vi "2DUniqueArraySet.vi"(10 "Colums":i32=6, 11 "Rows":i32=3) -> (0 "2D Double Array":i32[][](array[numeric]), 3 "2D String Array":string[][](array[string]))   [LabVIEW 2023]
uses:
  <vilib>/numeric/Random Number (Range) U64.vi
  <vilib>/numeric/sub_Random U32.vi
panel:
  # "Генерира 6 \"уникални\" числа.\n\"Унникалността\" се запазва единствено и само за елементите в колоните на даден ред,\n но не и между редовете."
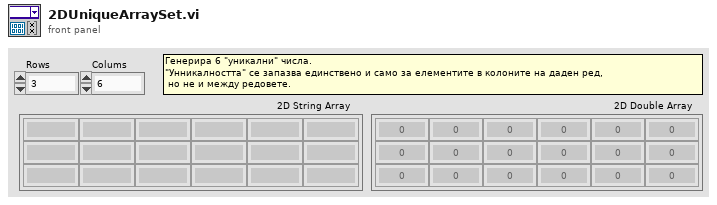
[diagram p1: front panel]
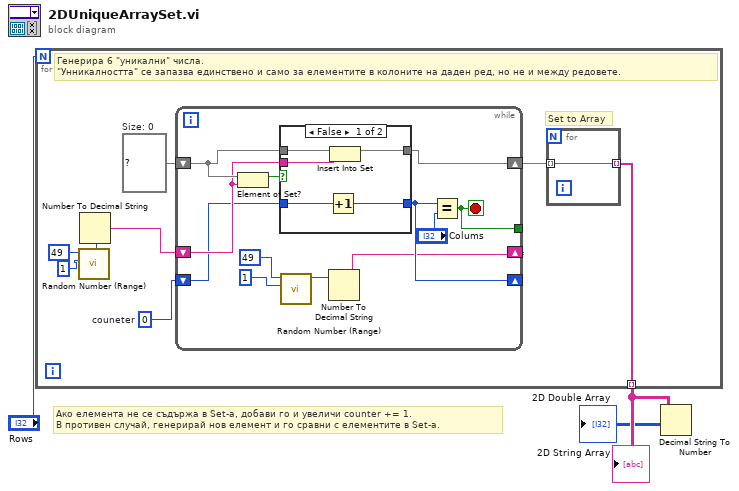
[diagram p0: block diagram]
diagram:
  # "Ако елемента не се съдържа в Set-а, добави го и увеличи counter += 1.\nВ противен случай, генерирай нов елемент и го сравни с елементите в Set-а."
  n1 = for {
    N: "Rows" -> [_]
    tunnel: [w5] -> w2 mode=indexing
    w4 = set{string} {}  # Size: 0
    w7 = 0  # couneter
    # "Генерира 6 \"уникални\" числа.\n\"Унникалността\" се запазва единствено и само за елементите в колоните на даден ред, но не и между редовете."
    # "Set to Array"
    n2 = call-poly <vilib>:"Random Number (Range).vi"("lower bound (0)"=u64 1, "upper bound (100)"=u64 49) -> ("number"=w11:u64)  [unwired: 9 in]
    n3 = Number To Decimal String(number=w11) -> (decimal integer string=w8:string)  [unwired: 1 in]
    n4 = while {
      shift-right: [w21] -> w6
      shift-left: w4 -> [w23]
      shift-right: [w14] -> _
      shift-left: w8 -> [w22]
      shift-right: [w19] -> _
      shift-left: w7 -> [w20]
      tunnel: [w13] -> _
      stop <- w13 stop-if-true
      n5 = Element of Set?(10:w22, 11:w23) -> (3:w24:bool)
      n6 = case shown="False" w24 {
        tunnel: w23 -> [w29 w31]
        tunnel: w22 -> [w27 _]
        tunnel: [w28 w31] -> w21
        tunnel: w20 -> [w26 w30]
        tunnel: [w25 w30] -> w19
        frame False {
          n7 = Increment(x=w26) -> (x+1=w25:i32)
          n8 = Insert Into Set(10:w27, 11:w29) -> (3:w28:set{string})  [unwired: 1 out]
        }
        frame True {
        }
      }
      n9 = call-poly <vilib>:"Random Number (Range).vi"("lower bound (0)"=u64 1, "upper bound (100)"=u64 49) -> ("number"=w17:u64)  [unwired: 9 in]
      n10 = Number To Decimal String(number=w17) -> (decimal integer string=w14:string)  [unwired: 1 in]
      n11 = Equal?(x=w19, y="Colums") -> (x = y?=w13:bool)
    }
    n12 = for {
      tunnel: [w12] -> w5 mode=indexing
      tunnel: w6 -> [w12] mode=indexing
    }
  }
  "2D String Array" <- w2
  n13 = Decimal String To Number(string=w2) -> (number=→"2D Double Array":i32[][])  [unwired: 2 in, 1 out]
